vi "Analyse_Error.vi"(0 "Error_Under_Analysis":errorcluster, 11 "Error_In":errorcluster) -> (4 "State_and_Data":T1, 15 "Error_Out":errorcluster)   [LabVIEW 2023]
uses:
  Controls/State_and_Data.ctl
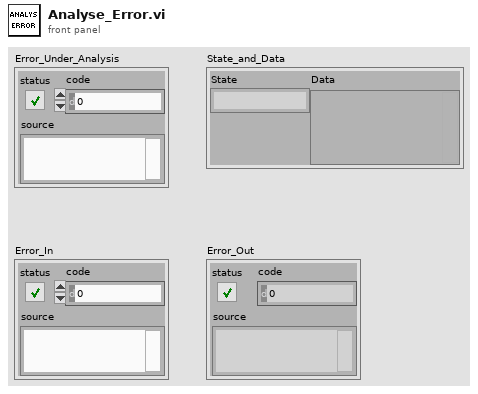
[diagram p1: front panel]
types:
  T1 = typedef "State_and_Data.ctl" = cluster{"State":string, "Data":variant}
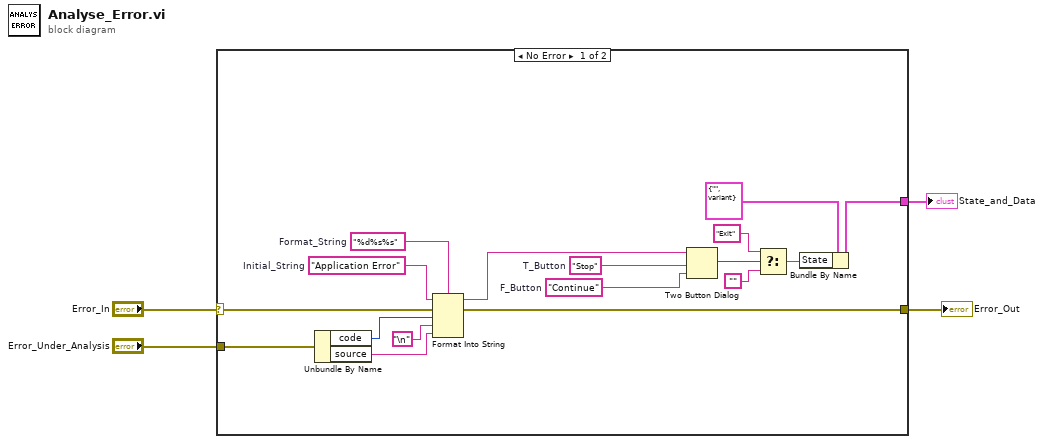
[diagram p0: block diagram]
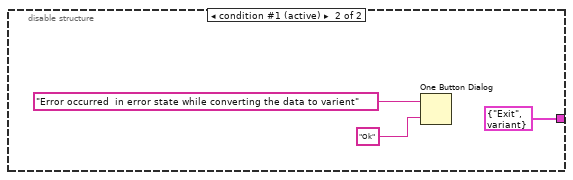
[diagram p3: hidden frame]
diagram:
  n1 = case shown="No Error" "Error_In" {
    selector: "Error_In" -> [w18 w23]
    tunnel: [w21 w22] -> w4
    tunnel: "Error_Under_Analysis" -> [w20 _]
    tunnel: [w19 w23] -> w2
    frame No Error {
      w10 = "%d%s%s"  # Format_String
      w9 = "Application Error"  # Initial_String
      w8 = "Stop"  # T_Button
      w7 = "Continue"  # F_Button
      n2 = Unbundle By Name(w20) -> ("code"=w12:i32, "source"=w13:string)
      n3 = Format Into String(format string=w10, initial string=w9, error in=w18, w12, "\n", w13) -> (resulting string=w6:string, error out=w19:errorcluster)
      n4 = Two Button Dialog(message=w6, 1:w7, 2:w8) -> (T button?=w15:bool)
      n5 = Select(t="Exit" ("State"), s=w15, f="") -> (s? t:f=w17:string)
      n6 = Bundle By Name(cluster=T1 {"State"="", "Data"=variant} ("State_and_Data"), "State"=w17) -> (w21:T1)
    }
    frame Error {
      n7 = disable-structure shown="RUN_TIME_ENGINE==True" {
        disable-tunnel: [_ T1 {"State"="Exit", "Data"=variant} ("State_and_Data")] -> w22
        frame condition #0 {
        }
        frame condition #1 (active) {
          n8 = One Button Dialog(message="Error occurred  in error state while converting the data to varient", button name ("OK")="Ok") -> ()  [unwired: 1 out]
        }
      }
    }
  }
  "State_and_Data" <- w4
  "Error_Out" <- w2
